vi "loadRfChannel.vi"(8 "error in (no error)":errorcluster, 9 "Channel.lvclass":refnum<class "Channel.lvclass">, 10 "xmlNode.lvclass":refnum<class "xmlNode.lvclass">, 11 "deviceDataBase in":refnum<class "deviceDataBase.lvclass">) -> (0 "error out":errorcluster, 1 "Channel.lvclass out":refnum<class "Channel.lvclass">, 2 "xmlNode out":refnum<class "xmlNode.lvclass">, 3 "deviceDataBase out":refnum<class "deviceDataBase.lvclass">)   [LabVIEW 2009, in "Tools.lvlib" / "DatabaseHelpers.lvlib" / "deviceDataBase.lvclass"]
uses:
  deviceDataBase.lvclass
  xmlNode/xmlNode.lvclass
  Database Objects/Channel/Channel.lvclass
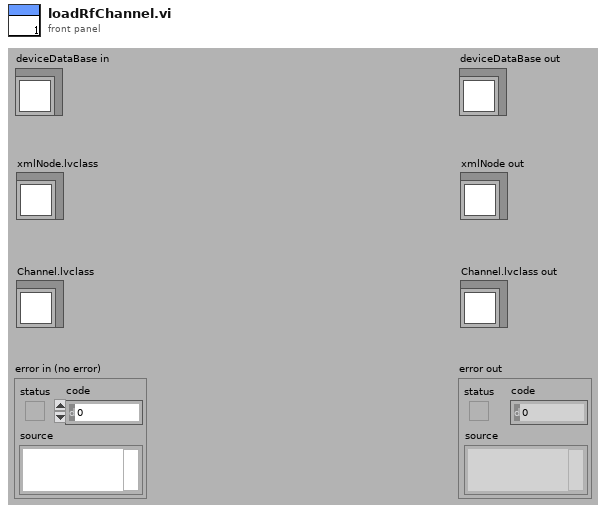
[diagram p1: front panel]
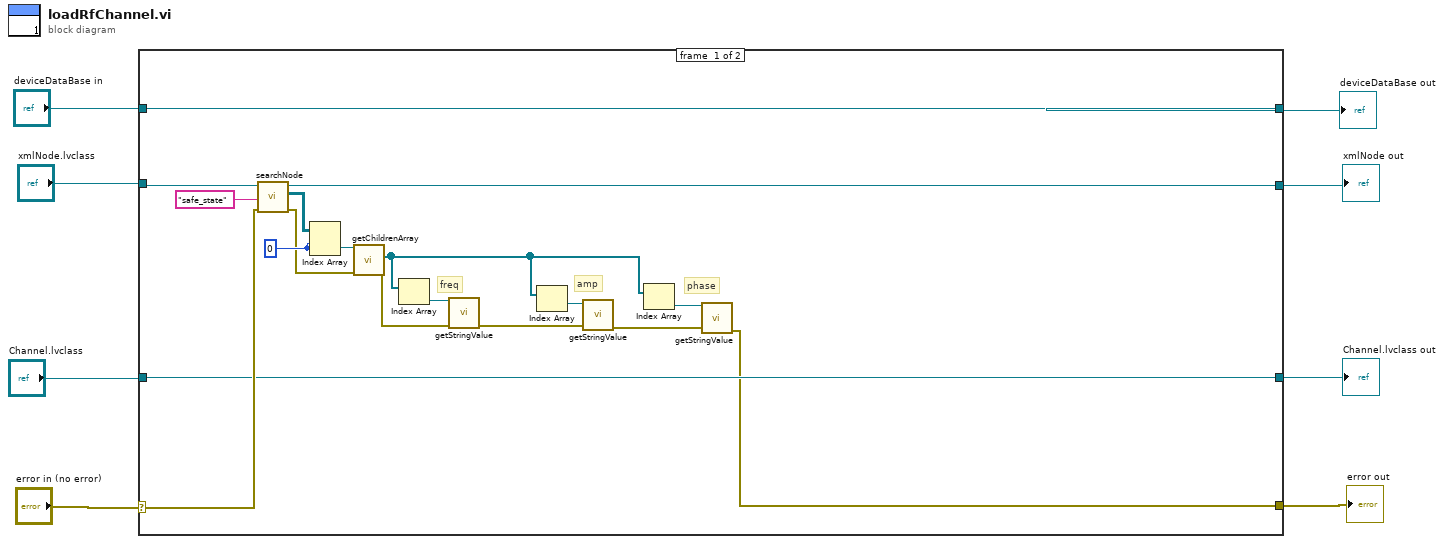
[diagram p0: block diagram]
diagram:
  n1 = case shown="No Error" "error in (no error)" {
    selector: "error in (no error)" -> [w17 w30]
    tunnel: [w11 w30] -> w7
    tunnel: [w26 w29] -> w5
    tunnel: "deviceDataBase in" -> [w26 w29]
    tunnel: "xmlNode.lvclass" -> [w18 w27]
    tunnel: "Channel.lvclass" -> [w12 w28]
    tunnel: [w16 w27] -> w2
    tunnel: [w12 w28] -> w1
    frame #0 {
      w23 = 0
      # "phase"
      # "amp"
      # "freq"
      n2 = call-dynamic "searchNode.vi"("error in (no error)"=w17, "searchElementName"="safe_state", "xmlNode in"=w18) -> ("error out"=w21:errorcluster, "arrayXmlNodes"=w24:refnum<class "xmlNode.lvclass">[][], "xmlNode out"=w16:refnum<class "xmlNode.lvclass">)  [unwired: 6 in]
      n3 = Index Array(array=w24, index (row)=w23, index (col)=w23) -> (element=w22:refnum<class "xmlNode.lvclass">)
      n4 = call-dynamic "getChildrenArray.vi"("error in (no error)"=w21, "xmlNode.lvclass in"=w22) -> ("error out"=w19:errorcluster, "Children"=w15:refnum<class "xmlNode.lvclass">[])  [unwired: 7 in, 1 out]
      n5 = Index Array(array=w15) -> (element=w20:refnum<class "xmlNode.lvclass">)  [unwired: 1 in]
      n6 = call-dynamic "getStringValue.vi"("error in (no error)"=w19, "xmlNode.lvclass in"=w20) -> ("error out"=w10:errorcluster)  [unwired: 7 in, 2 out]
      n7 = Index Array(array=w15) -> (element=w14:refnum<class "xmlNode.lvclass">)  [unwired: 1 in]
      n8 = call-dynamic "getStringValue.vi"("error in (no error)"=w10, "xmlNode.lvclass in"=w14) -> ("error out"=w9:errorcluster)  [unwired: 7 in, 2 out]
      n9 = Index Array(array=w15) -> (element=w13:refnum<class "xmlNode.lvclass">)  [unwired: 1 in]
      n10 = call-dynamic "getStringValue.vi"("error in (no error)"=w9, "xmlNode.lvclass in"=w13) -> ("error out"=w11:errorcluster)  [unwired: 7 in, 2 out]
    }
    frame #1 {
    }
  }
  "error out" <- w7
  "deviceDataBase out" <- w5
  "xmlNode out" <- w2
  "Channel.lvclass out" <- w1
